vi "Fit.vi"() -> ()   [LabVIEW 2017]
uses:
  <vilib>/Analysis/NI_AALPro.lvlib
panel:
  out "Formula":string
  out "Waveform Graph":dbl[][](graph)
  in  "Filtered X":dbl[](array[numeric])=[667.0, 667.0, 667.0, 667.0, 667.0, 667.0, 667.0, 667.0, 680.0, 680.0, 680.0, 680.0, 830.0, 680.0, 680.0, 680.0, 680.0, 689.0, 691.0, 692.0, 692.0, 692.0, 693.0, 693.0, 693.0, 693.0, 694.0, 695.0, 695.0, 696.0, 698.0, 699.0, 700.0, 701.0, 702.0, 704.0, 705.0, 710.0, 711.0, 712.0, 713.0, 715.0, 716.0, 718.0, 720.0, 721.0, 723.0, 724.0, 725.0, 726.0, 726.0, 727.0, 728.0, 729.0, 733.0, 735.0, 737.0, 739.0, 745.0, 747.0, 747.0, 747.0, 747.0, 747.0, 748.0, 749.0, 750.0, 751.0, 753.0, 754.0, 755.0, 756.0, 759.0, 762.0, 765.0, 766.0, 767.0, 769.0, 771.0, 774.0, 775.0, 775.0, 777.0, 777.0, 777.0, 778.0, 778.0, 778.0, 778.0, 778.0, 779.0, 779.0, 779.0, 779.0, 779.0, 779.0, 779.0, 779.0, 779.0, 760.0, 760.0, 760.0, 760.0, 745.0, 750.0, 750.0, 752.0, 752.0, 752.0, 752.0, 752.0, 752.0, 752.0, 752.0, 752.0, 752.0, 751.0, 749.0, 748.0, 747.0, 747.0, 746.0, 745.0, 745.0, 746.0, 746.0, 746.0, 746.0, 747.0, 748.0, 748.0, 748.0, 748.0, 748.0, 748.0, 748.0, 748.0, 748.0, 748.0, 748.0, 748.0, 748.0, 747.0, 747.0, 747.0, 747.0, 748.0, 749.0, 750.0, 751.0, 752.0, 753.0, 755.0, 757.0, 759.0, 760.0, 762.0, 763.0, 765.0, 765.0, 813.0, 817.0, 822.0, 824.0, 826.0, 835.0, 842.0, 843.0, 844.0, 846.0, 851.0, 851.0, 851.0, 852.0, 854.0, 856.0, 856.0, 857.0, 859.0, 861.0, 862.0, 862.0, 865.0, 871.0, 874.0, 877.0, 880.0, 881.0, 885.0, 886.0, 887.0, 887.0, 888.0, 890.0, 892.0, 893.0, 895.0, 897.0, 901.0, 912.0, 916.0, 918.0, 920.0, 923.0, 926.0, 930.0, 931.0, 936.0, 959.0, 963.0, 963.0, 963.0, 1063.0, 1067.0, 1070.0, 1073.0, 1076.0, 1079.0, 1081.0, 1084.0, 1087.0, 1089.0, 1093.0, 1096.0, 1102.0, 1106.0, 1110.0, 1113.0, 1114.0, 1117.0, 1118.0, 1120.0, 1121.0, 1125.0, 1131.0, 1136.0, 1138.0, 1143.0, 1145.0, 1147.0, 1148.0, 1150.0, 1151.0, 1157.0, 1160.0, 1164.0, 1167.0, 1169.0, 1172.0, 1176.0, 1177.0, 1182.0, 1185.0, 1188.0, 1196.0, 1204.0, 1205.0, 1206.0, 1211.0, 1214.0, 1220.0, 1222.0, 1226.0, 1234.0, 1238.0, 1242.0, 1248.0, 1253.0, 1253.0, 1259.0, 1278.0, 1283.0, 1283.0, 1284.0, 1284.0, 1284.0, 1284.0, 1284.0, 1290.0, 1293.0, 1294.0, 1303.0, 1313.0, 1321.0, 1334.0, 1350.0, 1355.0, 1356.0, 1360.0, 1361.0, 1363.0, 1363.0, 1363.0, 1366.0, 1367.0, 1368.0, 1373.0, 1377.0, 1381.0, 1388.0, 1393.0, 1402.0, 1406.0, 1410.0, 1419.0, 1430.0, 1438.0, 1460.0, 1460.0, 1460.0, 1460.0, 1460.0, 1460.0, 1460.0, 1460.0, 1460.0, 1457.0, 1457.0, 1503.0, 1508.0, 1514.0, 1521.0, 1539.0, 1561.0, 1566.0, 1573.0, 1577.0, 1581.0, 1581.0, 1583.0, 1583.0, 1583.0, 1604.0, 1617.0, 1621.0, 1625.0, 1629.0, 1629.0, 1637.0, 1639.0, 1643.0, 1655.0, 1680.0, 1685.0, 1695.0, 1706.0, 1706.0, 1706.0, 1706.0, 1706.0, 1713.0, 1724.0, 1744.0, 1760.0, 1770.0, 1779.0, 1781.0, 1781.0, 1784.0, 1786.0, 1786.0, 1786.0, 1786.0, 1863.0, 1877.0, 1879.0, 1890.0, 1895.0, 1895.0, 1895.0, 1903.0, 1903.0, 1903.0, 1903.0, 1903.0, 1903.0, 1903.0, 1903.0, 1903.0, nan, 700.0, 701.0, 701.0, 701.0, 701.0, 701.0, 701.0, 701.0, 701.0, 701.0, 701.0, 700.0, 700.0, 700.0, 700.0, 700.0, 700.0, 700.0, 699.0, 697.0, 695.0, 695.0, 695.0, 693.0, 693.0, 693.0, 692.0, 692.0, 691.0, 691.0, 691.0, 691.0, 690.0, 688.0, 686.0, 684.0, 683.0, 683.0, 683.0, 683.0, 683.0, 682.0, 681.0, 680.0, 679.0, 679.0, 678.0, 678.0, 677.0, 676.0, 675.0, 674.0, 674.0, 674.0, 674.0, 674.0, 674.0, 674.0, 674.0, 674.0, 672.0, 671.0, 669.0, 669.0, 668.0, 668.0, 668.0, 667.0, 666.0, 666.0, 666.0, 665.0, 665.0, 665.0, 665.0, 664.0, 663.0, 663.0, 663.0, 661.0, 661.0, 661.0, 661.0, 661.0, 661.0, 661.0, 661.0, 661.0]
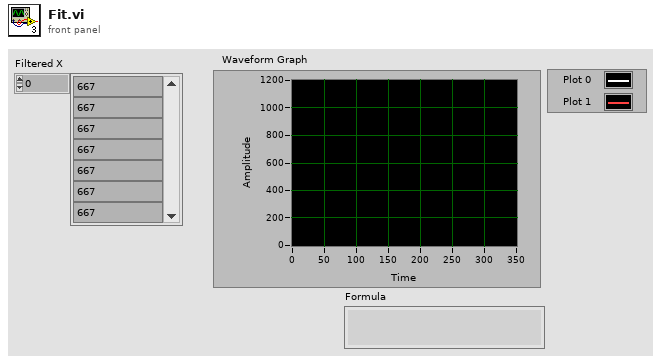
[diagram p1: front panel]
types:
  T1 = enum16{"Linear", "Polynomial", "Exponential", "Power"}
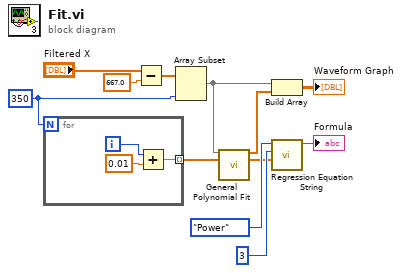
[diagram p0: block diagram]
diagram:
  w11 = 350 ("length")
  n1 = for {
    N: w11 -> [_]
    tunnel: [w14] -> w6 mode=indexing
    i -> [w15]
    n2 = Add(x=w15, y=0.01) -> (x+y=w14:dbl)
  }
  n3 = Subtract(x="Filtered X", y=667.0) -> (x-y=w2:dbl[])
  n4 = Array Subset(array=w2, length=w11) -> (w7:dbl[])  [unwired: 1 in]
  n5 = call <vilib>:"General Polynomial Fit.vi"("Y"=w7, "X"=w6) -> ("Best Polynomial Fit"=w5:dbl[], "Polynomial Coefficients"=w4:dbl[])  [unwired: 10 in, 2 out]
  n6 = Build Array(w7, w5) -> (→"Waveform Graph":dbl[][])
  n7 = call "Regression Equation String.vi"("coefficients"=w4, "precision"=3, "fit type"=T1."Power") -> ("Formula"=→"Formula":string)  [unwired: 8 in]
